vi "AckRequest.vi"(8 "error in (no error)":errorcluster, 10 "RUID":string, 11 "PUID":string) -> (0 "error out":errorcluster, 2 "Response":string)   [LabVIEW 2015, in "PersonnelRestApi.lvlib"]
uses:
  PersonnelRestApi.lvlib
  TypeDef/PostPersonnelCommands.ctl
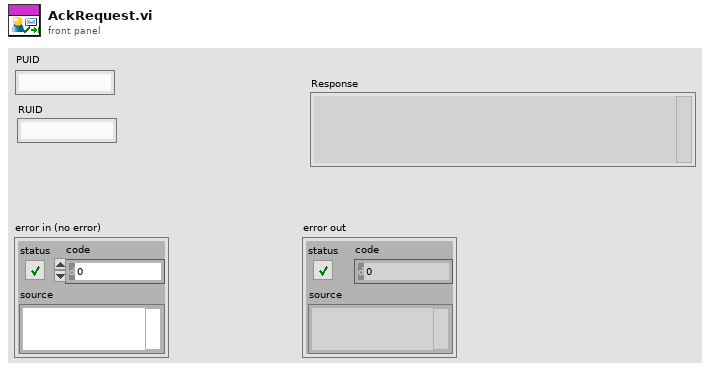
[diagram p1: front panel]
types:
  T1 = typedef "PersonnelRestApi.lvlib/PostPersonnelCommands.ctl" = enum16{"WriteRole", "WriteName", "AddRequest", "RemoveRequest", "IntoRoom", "OutOfRoom", "Register", "AckRequest"}
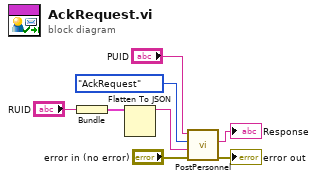
[diagram p0: block diagram]
diagram:
  n1 = Bundle("RUID"="RUID") -> (w2:cluster{"RUID":string})  [unwired: 1 in]
  n2 = Flatten To JSON(anything=w2) -> (JSON string=w1:string)  [unwired: 2 in, 1 out]
  n3 = call "PostPersonnel.vi"("error in (no error)"="error in (no error)", "Data"=w1, "Commands"=PostPersonnelCommands."AckRequest", "PUID"="PUID") -> ("error out"=→"error out":errorcluster, "body"=→"Response":string)  [unwired: 6 in]
